vi "PH_Beckhoff_PP_PU.handle PSU DAs.vi"(0 "i ref in":refnum<vi>, 2 "Digital Output Values":T1, 3 "Changed digital Outputs":i32[](array[numeric]), 5 "error in":errorcluster) -> (14 "i ref out":refnum<vi>, 19 "error out":errorcluster)   [LabVIEW 2014, in "PH_Beckhoff_PP_PU.lvlib"]
uses:
  PH_Beckhoff_PP_PU.lvlib
  PH_Beckhoff/PH_Beckhoff.Digital Outputs.ctl
  PH_Beckhoff/PH_Beckhoff.lvlib
  PH_Common/PH_Common.lvlib
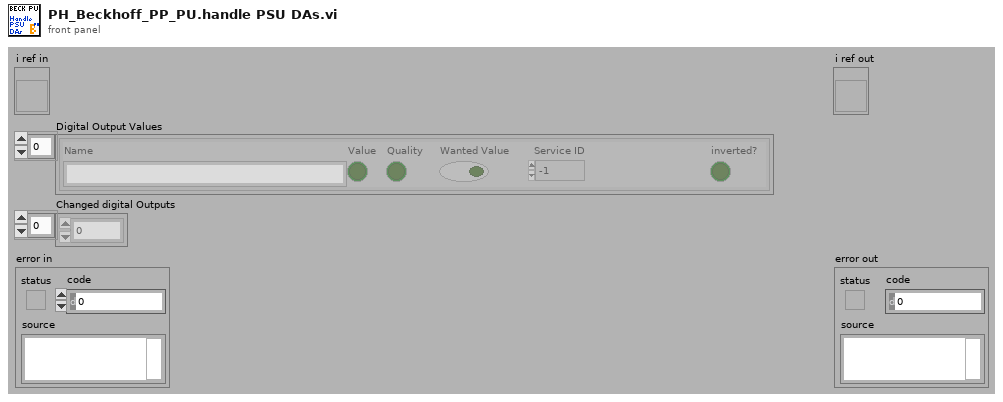
[diagram p1: front panel]
types:
  T1 = typedef "PH_Beckhoff.lvlib/PH_Beckhoff.Digital Outputs.ctl" = cluster{"Name":string, "Value":bool, "Quality":bool, "Wanted Value":bool, "Service ID":i32, "inverted?":bool}[]
  T2 = typedef "PH_Beckhoff_PP_PU.lvlib/PH_Beckhoff_PP_PU.i attribute.ctl" = cluster{"HV Meas":cluster{"Input GUI Ref":refnum<vi>, "Voltage Service ID":i32, "Voltage [V]":dbl, "Quality":bool, "# in Data":i32}[], "Trigger":cluster{"Status":cluster{"GUI Ref":refnum<vi>, "Status Service ID":i32, "Status":T3}, "last shot:":cluster{"GUI Ref":refnum<vi>, "Service ID":i32, "Time":string}, "DIs":cluster{"triggered":cluster{"GUI Ref":refnum<vi>, "# in Data":i32}, "fired":cluster{"GUI Ref":refnum<vi>, "# in Data":i32}}, "GUI Ref Indicator":refnum<vi>}[], "RR":cluster{"Status":cluster{"GUI Ref":refnum<vi>, "Status Service ID":i32, "Status":T3}, "DIs":cluster{"closed":cluster{"GUI Ref":refnum<vi>, "# in Data":i32}, "open":cluster{"GUI Ref":refnum<vi>, "# in Data":i32}}, "Close":cluster{"GUI Ref":refnum<vi>, "# in Data":i32}, "GUI Ref Indicator":refnum<vi>}[], "Igni":cluster{"Status":cluster{"GUI Ref":refnum<vi>, "Status Service ID":i32, "Status":T3}, "DIs":cluster{"heating on":cluster{"GUI Ref":refnum<vi>, "# in Data":i32}, "water on":cluster{"GUI Ref":refnum<vi>, "# in Data":i32}}, "Device on":cluster{"GUI Ref":refnum<vi>, "# in Data":i32}, "GUI Ref Indicator":refnum<vi>}[], "PSU":cluster{"Status":cluster{"GUI Ref":refnum<vi>, "Status Service ID":i32, "Status":T3}, "Limit Service ID":i32, "DIs":cluster{"inhibit":cluster{"GUI Ref":refnum<vi>, "# in Data":i32}, "end of charge":cluster{"GUI Ref":refnum<vi>, "# in Data":i32}, "HV on":cluster{"GUI Ref":refnum<vi>, "# in Data":i32}, "overtemp":cluster{"GUI Ref":refnum<vi>, "# in Data":i32}, "interlock":cluster{"GUI Ref":refnum<vi>, "# in Data":i32}, "load fault":cluster{"GUI Ref":refnum<vi>, "# in Data":i32}, "sum fault":cluster{"GUI Ref":refnum<vi>, "# in Data":i32}, "HV off":cluster{"GUI Ref":refnum<vi>, "# in Data":i32}, "DC ok":cluster{"GUI Ref":refnum<vi>, "# in Data":i32}}, "AIs":cluster{"voltage":cluster{"GUI Ref":refnum<vi>, "# in Data":i32}, "current":cluster{"GUI Ref":refnum<vi>, "# in Data":i32}}, "DAs":cluster{"inhibit":cluster{"GUI Ref":refnum<vi>, "# in Data":i32}, "interlock":cluster{"GUI Ref":refnum<vi>, "# in Data":i32}, "HV on":cluster{"GUI Ref":refnum<vi>, "# in Data":i32}, "Reset":cluster{"GUI Ref":refnum<vi>, "# in Data":i32}}, "AAs":cluster{"Voltage to set":cluster{"GUI Ref":refnum<vi>, "# in Data":i32}}, "GUI Ref Indicator":refnum<vi>}[], "reconfigured":cluster{"?":bool, "GUI Ref":refnum<vi>}, "PU Rack Type":T4, "HV Meas Info":T5, "PSU Info":T6}
  T3 = typedef "PH_StatusHandler.lvlib/PH_StatusHandler.Status.ctl" = i16
  T4 = typedef "PH_Beckhoff_PP_PU.lvlib/PH_Beckhoff_PP_PU.PU Rack Type.ctl" = enum16{"no Info", "PA 19mm", "PA 45mm", "MA PU 1 and 2", "MA PU 3 and 4", "MA PU 5 and 6", "MA FR and PILC"}
  T5 = typedef "PH_Beckhoff_PP_PU.lvlib/PH_Beckhoff_PP_PU.HV Meas Info.ctl" = cluster{"Period Time [s]":dbl, "Subtractor 1 [Hz]":dbl, "Devider 1 [Hz/kV]":dbl, "Subtractor 2 [Hz]":dbl, "Devider 2 [Hz/kV]":dbl}
  T6 = typedef "PH_Beckhoff_PP_PU.lvlib/PH_Beckhoff_PP_PU.PSU Info.ctl" = cluster{"Limits 1 [V]":cluster{"Lower":dbl, "Upper":dbl}, "Limits 2 [V]":cluster{"Lower":dbl, "Upper":dbl}}
  T7 = cluster{"Status":cluster{"GUI Ref":refnum<vi>, "Status Service ID":i32, "Status":T3}, "Limit Service ID":i32, "DIs":cluster{"inhibit":cluster{"GUI Ref":refnum<vi>, "# in Data":i32}, "end of charge":cluster{"GUI Ref":refnum<vi>, "# in Data":i32}, "HV on":cluster{"GUI Ref":refnum<vi>, "# in Data":i32}, "overtemp":cluster{"GUI Ref":refnum<vi>, "# in Data":i32}, "interlock":cluster{"GUI Ref":refnum<vi>, "# in Data":i32}, "load fault":cluster{"GUI Ref":refnum<vi>, "# in Data":i32}, "sum fault":cluster{"GUI Ref":refnum<vi>, "# in Data":i32}, "HV off":cluster{"GUI Ref":refnum<vi>, "# in Data":i32}, "DC ok":cluster{"GUI Ref":refnum<vi>, "# in Data":i32}}, "AIs":cluster{"voltage":cluster{"GUI Ref":refnum<vi>, "# in Data":i32}, "current":cluster{"GUI Ref":refnum<vi>, "# in Data":i32}}, "DAs":cluster{"inhibit":cluster{"GUI Ref":refnum<vi>, "# in Data":i32}, "interlock":cluster{"GUI Ref":refnum<vi>, "# in Data":i32}, "HV on":cluster{"GUI Ref":refnum<vi>, "# in Data":i32}, "Reset":cluster{"GUI Ref":refnum<vi>, "# in Data":i32}}, "AAs":cluster{"Voltage to set":cluster{"GUI Ref":refnum<vi>, "# in Data":i32}}, "GUI Ref Indicator":refnum<vi>}[]
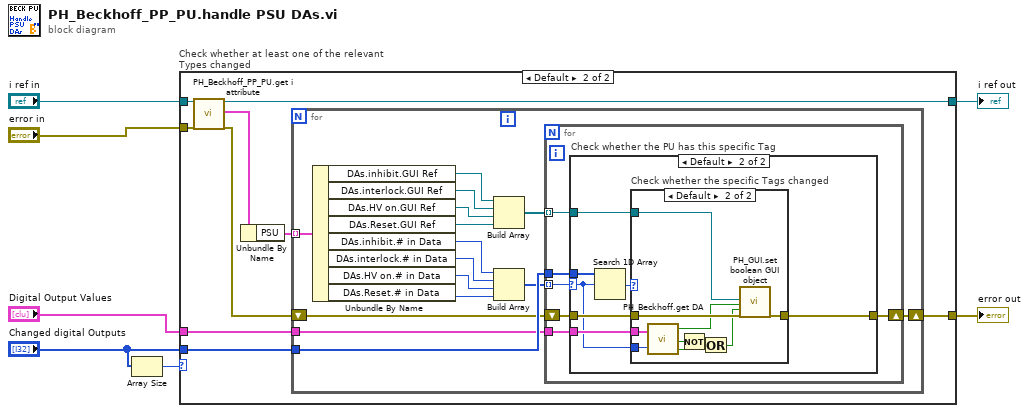
[diagram p0: block diagram]
diagram:
  n1 = Array Size(array="Changed digital Outputs") -> (size(s)=w1:i32)
  n2 = case "Check whether at least one of the relevant Types changed" shown="Default" w1 {
    tunnel: "error in" -> [w9 w15]
    tunnel: [w9 w18] -> w7
    tunnel: "Digital Output Values" -> [_ w17]
    tunnel: "Changed digital Outputs" -> [_ w16]
    tunnel: [w8 w13] -> w4
    tunnel: "i ref in" -> [w8 w12]
    frame 0 {
    }
    frame Default {
      n3 = call "PH_Beckhoff_PP_PU.get i attribute.vi"("i ref in"=w12, "error in (no error)"=w15) -> ("i ref out"=w13:refnum<vi>, "i attribute"=w11:T2, "error out"=w14:errorcluster)  [unwired: 15 in]
      n4 = Unbundle By Name(w11) -> ("PSU"=w10:T7)
      n5 = for {
        tunnel: w17 -> [w19]
        tunnel: w16 -> [w32]
        shift-right: [w33] -> w18
        shift-left: w14 -> [w31]
        tunnel: w10 -> [w30] mode=indexing
        n6 = Unbundle By Name(w30) -> ("DAs.inhibit.GUI Ref"=w26:refnum<vi>, "DAs.interlock.GUI Ref"=w27:refnum<vi>, "DAs.HV on.GUI Ref"=w28:refnum<vi>, "DAs.Reset.GUI Ref"=w29:refnum<vi>, "DAs.inhibit.# in Data"=w22:i32, "DAs.interlock.# in Data"=w23:i32, "DAs.HV on.# in Data"=w24:i32, "DAs.Reset.# in Data"=w25:i32)
        n7 = Build Array(w26, w27, w28, w29) -> (w21:refnum<vi>[])
        n8 = Build Array(w22, w23, w24, w25) -> (w20:i32[])
        n9 = for {
          tunnel: w19 -> [w37]
          tunnel: w21 -> [w36] mode=indexing
          tunnel: w20 -> [w35] mode=indexing
          tunnel: w32 -> [w34]
          shift-right: [w38] -> w33
          shift-left: w31 -> [w39]
          n10 = case "Check whether the PU has this specific Tag" shown="Default" w35 {
            selector: w35 -> [_ w43]
            tunnel: w39 -> [w40 w47]
            tunnel: [w40 w46] -> w38
            tunnel: w37 -> [_ w45]
            tunnel: w36 -> [_ w44]
            tunnel: w34 -> [_ w42]
            frame -1 {
            }
            frame Default {
              n11 = Search 1D Array(1D array=w42, element=w43) -> (index of element=w41:i32)  [unwired: 1 in]
              n12 = case "Check whether the specific Tags changed" shown="Default" w41 {
                tunnel: w47 -> [w48 w58]
                tunnel: [w48 w57] -> w46
                tunnel: w45 -> [_ w49]
                tunnel: w44 -> [_ w56]
                tunnel: w43 -> [_ w50]
                frame -1 {
                }
                frame Default {
                  n13 = call "PH_Beckhoff.get DA.vi"("Digital Outputs"=w49, "index of element"=w50) -> ("Value"=w55:bool, "Quality"=w52:bool, "Tag not found"=w53:bool)
                  n14 = Not(x=w52) -> (.not. x?=w51:bool)
                  n15 = Or(x=w51, y=w53) -> (x .or. y?=w54:bool)
                  n16 = call "PH_GUI.set boolean GUI object.vi"("Boolean Knob GUI Ref"=w56, "Value"=w55, "Blinking? (false)"=w54, "error in (no error)"=w58) -> ("error out"=w57:errorcluster)  [unwired: 15 in]
                }
              }
            }
          }
        }
      }
    }
  }
  "error out" <- w7
  "i ref out" <- w4
